vi "MTS_GetFileFromWS.vi"(9 "File No":i32=-1, 10 "Tree Label":string, 11 ".pt3 File Name":path) -> (2 "File Header":T1, 3 "File Found":bool)   [LabVIEW 2013]
uses:
  Controls/Control.ctl
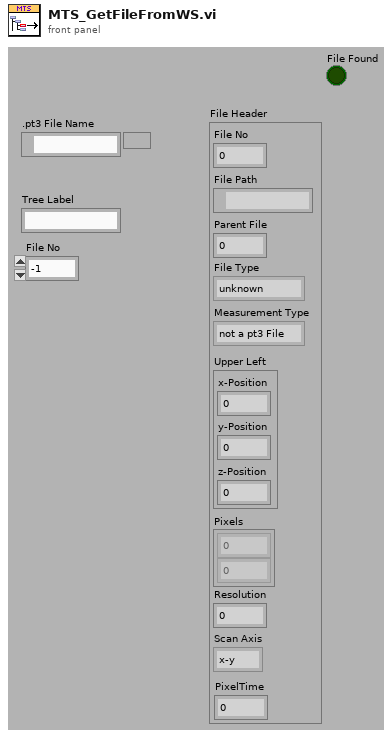
[diagram p1: front panel]
types:
  T1 = cluster{"File No":i32, "File Path":path, "Parent File":i32, "File Type":enum16{"unknown", "pt3 File", "png Image", "bmp Image"}, "Measurement Type":enum16{"not a pt3 File", "Image File", "Point Measurement", "Auto Point", "Line Scan", "Grid Scan"}, "Upper Left":cluster{"x-Position":dbl, "y-Position":dbl, "z-Position":dbl}, "Pixels":i32[], "Scan Axis":enum32{"x-y", "x-z", "y-z"}, "Resolution":dbl, "PixelTime":dbl}
  T2 = typedef "Control.ctl" = cluster{"File No":i32, "File Path":path, "Parent File":i32, "File Type":enum16{"unknown", "pt3 File", "png Image", "bmp Image"}, "Measurement Type":enum16{"not a pt3 File", "Image File", "Point Measurement", "Auto Point", "Line Scan", "Grid Scan"}, "Upper Left":cluster{"x-Position":dbl, "y-Position":dbl, "z-Position":dbl}, "Pixels":i32[], "Scan Axis":enum32{"x-y", "x-z", "y-z"}, dbl, dbl}
  T3 = enum16{"Get (Default)", "Set Workspace", "Append File", "Change Comment"}
  T4 = cluster{"File No":i32, "File Path":path, "Parent File":i32, "File Type":enum16{"unknown", "pt3 File", "png Image", "bmp Image"}, "Measurement Type":enum16{"not a pt3 File", "Image File", "Point Measurement", "Auto Point", "Line Scan", "Grid Scan"}, "Upper Left":cluster{"x-Position":dbl, "y-Position":dbl, "z-Position":dbl}, "Pixels":i32[], "Scan Axis":enum32{"x-y", "x-z", "y-x", "y-z", "z-x", "z-y"}, "Resolution":dbl, "PixelTime":dbl}[]
  T5 = cluster{"File No":i32, "File Path":path, "Parent File":i32, "File Type":enum16{"unknown", "pt3 File", "png Image", "bmp Image"}, "Measurement Type":enum16{"not a pt3 File", "Image File", "Point Measurement", "Auto Point", "Line Scan", "Grid Scan"}, "Upper Left":cluster{"x-Position":dbl, "y-Position":dbl, "z-Position":dbl}, "Pixels":i32[], "Scan Axis":u32, "Resolution":dbl, "PixelTime":dbl}
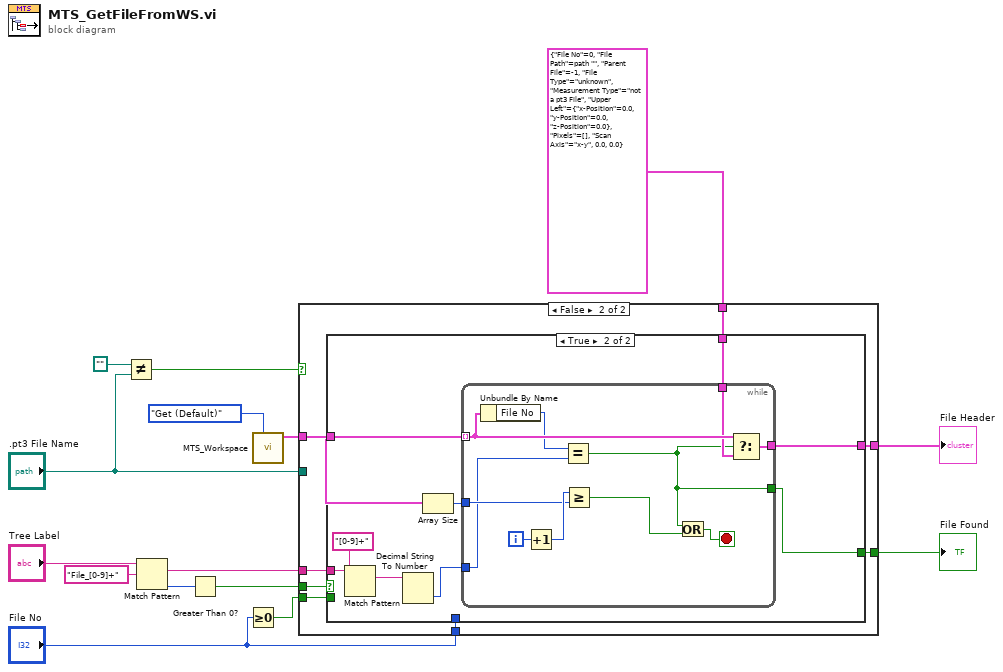
[diagram p0: block diagram]
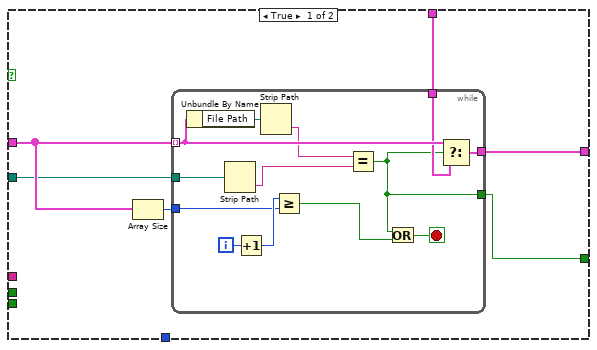
[diagram p2: hidden frame]
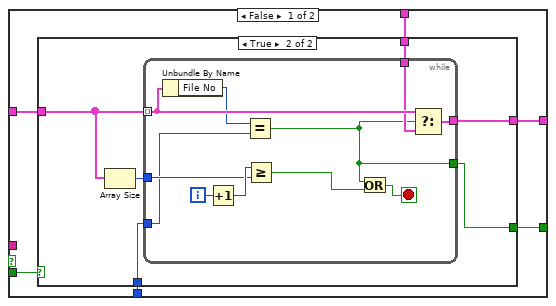
[diagram p3: hidden frame]
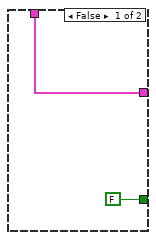
[diagram p4: hidden frame]
diagram:
  n1 = Not Equal?(x=path "", y=".pt3 File Name") -> (x != y?=w8:bool)
  n2 = Match Pattern(string="Tree Label", regular expression="File_[0-9]+") -> (match substring=w3:string, offset past match=w5:i32)  [unwired: 1 in, 2 out]
  n3 = Greater Than 0?(x=w5) -> (x > 0?=w4:bool)
  n4 = Greater Or Equal To 0?(x="File No") -> (x >= 0?=w2:bool)
  n5 = call "MTS_Workspace.vi"("Operation"=T3."Get (Default)") -> ("Files in Workspace"=w14:T4)  [unwired: 7 in, 3 out]
  n6 = case shown="False" w8 {
    tunnel: [w21 w42] -> w15
    tunnel: w14 -> [w19 w41]
    tunnel: T2 {"File No"=0, "File Path"=path "", "Parent File"=-1, "File Type"=enum."unknown", "Measurement Type"=enum."not a pt3 File", "Upper Left"={"x-Position"=0.0, "y-Position"=0.0, "z-Position"=0.0}, "Pixels"=[], "Scan Axis"=enum."x-y", 0.0, 0.0} ("f") -> [w18 w40]
    tunnel: [w17 w39] -> w11
    tunnel: ".pt3 File Name" -> [w16 _]
    tunnel: w4 -> [_ w38]
    tunnel: w3 -> [_ w37]
    tunnel: w2 -> [_ w36]
    tunnel: "File No" -> [_ w35]
    frame True {
      n7 = Array Size(array=w19) -> (size(s)=w20:i32)
      n8 = while {
        tunnel: w19 -> [w29] mode=indexing
        tunnel: w16 -> [w26]
        tunnel: w20 -> [w32]
        tunnel: [w28] -> w21
        tunnel: w18 -> [w23]
        tunnel: [w22] -> w17
        i -> [w34]
        stop <- w30 stop-if-true
        n9 = Unbundle By Name(w29) -> ("File Path"=w27:path)
        n10 = Strip Path(path=w26) -> (name=w24:string)  [unwired: 1 out]
        n11 = Increment(x=w34) -> (x+1=w33:i32)
        n12 = Strip Path(path=w27) -> (name=w25:string)  [unwired: 1 out]
        n13 = Greater Or Equal?(x=w33, y=w32) -> (x >= y?=w31:bool)
        n14 = Equal?(x=w25, y=w24) -> (x = y?=w22:bool)
        n15 = Or(x=w22, y=w31) -> (x .or. y?=w30:bool)
        n16 = Select(t=w29, s=w22, f=w23) -> (s? t:f=w28:T5)
      }
    }
    frame False {
      n17 = case shown="True" w38 {
        tunnel: [w47 w76] -> w42
        tunnel: w41 -> [w45 w74]
        tunnel: w40 -> [w46 w73]
        tunnel: [w48 w72] -> w39
        tunnel: w37 -> [_ w71]
        tunnel: w36 -> [w44 _]
        tunnel: w35 -> [w43 _]
        frame False {
          n18 = case shown="True" w44 {
            tunnel: [FALSE w51] -> w48
            tunnel: [w49 w54] -> w47
            tunnel: w46 -> [w49 w55]
            tunnel: w45 -> [_ w53]
            tunnel: w43 -> [_ w52]
            frame False {
            }
            frame True {
              n19 = Array Size(array=w53) -> (size(s)=w56:i32)
              n20 = while {
                tunnel: w53 -> [w62] mode=indexing
                tunnel: w56 -> [w65]
                tunnel: [w61] -> w54
                tunnel: w55 -> [w60]
                tunnel: [w57] -> w51
                tunnel: w52 -> [w58]
                i -> [w67]
                stop <- w63 stop-if-true
                n21 = Unbundle By Name(w62) -> ("File No"=w59:i32)
                n22 = Increment(x=w67) -> (x+1=w66:i32)
                n23 = Equal?(x=w59, y=w58) -> (x = y?=w57:bool)
                n24 = Greater Or Equal?(x=w66, y=w65) -> (x >= y?=w64:bool)
                n25 = Or(x=w57, y=w64) -> (x .or. y?=w63:bool)
                n26 = Select(t=w62, s=w57, f=w60) -> (s? t:f=w61:T5)
              }
            }
          }
        }
        frame True {
          n27 = Match Pattern(string=w71, regular expression="[0-9]+") -> (match substring=w69:string)  [unwired: 1 in, 3 out]
          n28 = Decimal String To Number(string=w69) -> (number=w68:i32)  [unwired: 2 in, 1 out]
          n29 = Array Size(array=w74) -> (size(s)=w75:i32)
          n30 = while {
            tunnel: w74 -> [w82] mode=indexing
            tunnel: w75 -> [w85]
            tunnel: [w81] -> w76
            tunnel: w73 -> [w80]
            tunnel: [w77] -> w72
            tunnel: w68 -> [w78]
            i -> [w87]
            stop <- w83 stop-if-true
            n31 = Unbundle By Name(w82) -> ("File No"=w79:i32)
            n32 = Increment(x=w87) -> (x+1=w86:i32)
            n33 = Equal?(x=w79, y=w78) -> (x = y?=w77:bool)
            n34 = Greater Or Equal?(x=w86, y=w85) -> (x >= y?=w84:bool)
            n35 = Or(x=w77, y=w84) -> (x .or. y?=w83:bool)
            n36 = Select(t=w82, s=w77, f=w80) -> (s? t:f=w81:T5)
          }
        }
      }
    }
  }
  "File Header" <- w15
  "File Found" <- w11
